vi "Proceed.vi"(7 "component is ready (Y)":bool=TRUE, 8 "error in (no error)":errorcluster, 10 "ProceedMessage":refnum<class "ProceedMessage.lvclass">, 11 "Retiga in":refnum<class "Retiga.lvclass">) -> (0 "error out":errorcluster, 2 "all observers are ready?":bool, 3 "Retiga out":refnum<class "Retiga.lvclass">)   [LabVIEW 2012, in "Retiga.lvclass"]
doc: "The Proceed method is used to check if your component is ready. Also it checks if the observers are ready. When the observers and the component are ready, it sends the proceed to its observee. If it's the highest observee, it distributes a stop command."
uses:
  Retiga.lvclass
  <vilib>/Distrio/Murmex/ProceedMessage/ProceedMessage.lvclass
  Retiga.lvclass/Retiga.ctl
  <vilib>/Distrio/Murmex/GenericMessage/GenericMessage.lvclass
  <vilib>/Distrio/Murmex/Murmex/Murmex.lvclass
  <vilib>/Distrio/Murmex/Message/Add or replace parameter.vi
  <vilib>/Distrio/Murmex/Message/Message.lvclass
  <vilib>/vision/NI_Vision_Development_Module.lvlib
panel:
  out "loop time (ms)":u32
  # "This method is called when the PROCEED\ntrigger is sent. \n\nOverride this method when your component needs to\nrespond to this trigger. \n\nCall parent for proper implementation"
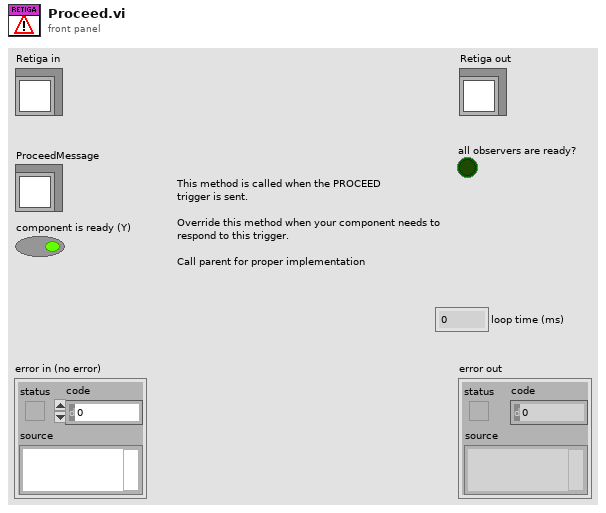
[diagram p1: front panel]
types:
  T1 = typedef "IMAQ Image.ctl" = refnum<image>
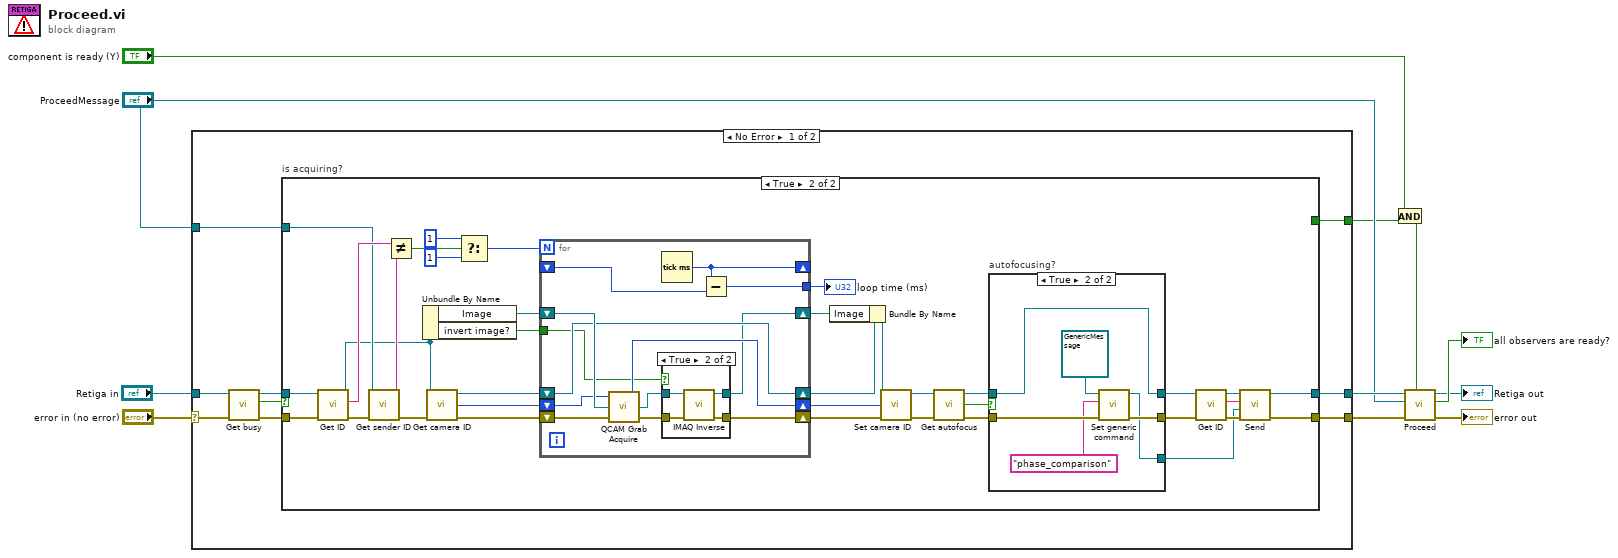
[diagram p0: block diagram]
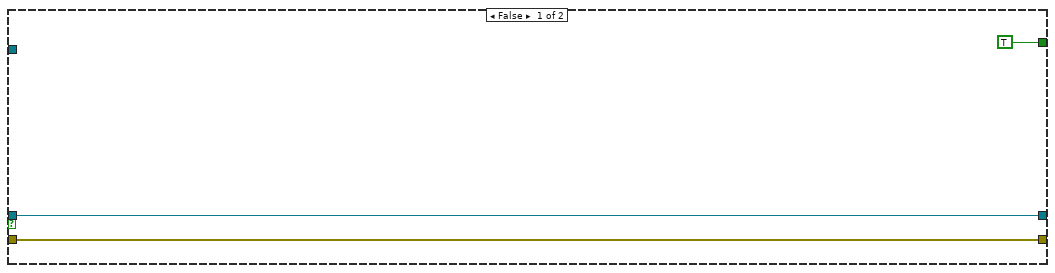
[diagram p2: hidden frame]
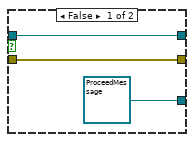
[diagram p3: hidden frame]
diagram:
  n1 = case shown="No Error" "error in (no error)" {
    selector: "error in (no error)" -> [w20 w89]
    tunnel: [w14 w89] -> w6
    tunnel: [w15 w88] -> w5
    tunnel: "Retiga in" -> [w19 w88]
    tunnel: "ProceedMessage" -> [w13 _]
    tunnel: [w12 _] -> w1
    frame No Error {
      n2 = call-dynamic "Get busy.vi"("error in (no error)"=w20, "Retiga in"=w19) -> ("error out"=w17:errorcluster, "busy?"=w18:bool, "Retiga out"=w16:refnum<class "Retiga.lvclass">)  [unwired: 7 in]
      n3 = case "is acquiring?" shown="True" w18 {
        tunnel: w17 -> [w22 w56]
        tunnel: w16 -> [w23 w55]
        tunnel: [w23 w27] -> w15
        tunnel: [w22 w26] -> w14
        tunnel: w13 -> [_ w54]
        tunnel: [TRUE _] -> w12
        frame False {
        }
        frame True {
          n4 = call <vilib>:"Get ID.vi"("error in (no error)"=w56, "Murmex in"=w55) -> ("error out"=w59:errorcluster, "component id"=w58:string, "Murmex out"=w48:refnum<class "Retiga.lvclass">)  [unwired: 7 in]
          n5 = call <vilib>:"Get sender ID.vi"("error in (no error)"=w59, "Message in"=w54) -> ("error out"=w49:errorcluster, "sender"=w57:string)  [unwired: 7 in, 1 out]
          n6 = Not Equal?(x=w58, y=w57) -> (x != y?=w51:bool)
          n7 = Unbundle By Name(w48) -> ("Image"=w44:T1, "invert image?"=w24:bool)
          n8 = call-dynamic "Get camera ID.vi"("error in (no error)"=w49, "Retiga in"=w48) -> ("error out"=w46:errorcluster, "camera ID"=w45:u32, "Retiga out"=w47:refnum<class "Retiga.lvclass">)  [unwired: 7 in]
          n9 = Select(t=1, s=w51, f=1) -> (s? t:f=w50:i32)
          n10 = for {
            N: w50 -> [_]
            shift-right: [w77] -> w43
            shift-left: w47 -> [w77]
            shift-right: [w75] -> w40
            shift-left: w46 -> [w81]
            shift-right: [w78] -> w39
            shift-left: w45 -> [w79]
            shift-right: [w73] -> w42
            shift-left: w44 -> [w80]
            shift-right: [w71] -> _
            shift-left: _ -> [w72]
            tunnel: [w70] -> w25
            tunnel: w24 -> [w69]
            n11 = call <userlib>:"QCAM Grab Acquire.vi"("error in (no error)"=w81, "Image"=w80, "cameraId"=w79) -> ("error out"=w76:errorcluster, "Image Out"=w74:T1, "cameraId out"=w78:u32)
            n12 = Tick Count (ms)() -> (millisecond timer value=w71:u32)
            n13 = case shown="True" w69 {
              tunnel: w76 -> [w82 w87]
              tunnel: [w82 w86] -> w75
              tunnel: w74 -> [w83 w85]
              tunnel: [w83 w84] -> w73
              frame False {
              }
              frame True {
                n14 = call "IMAQ Inverse"("error in (no error)"=w87, "Image Src"=w85) -> ("error out"=w86:errorcluster, "Image Dst Out"=w84:T1)  [unwired: 8 in]
              }
            }
            n15 = Subtract(x=w71, y=w72) -> (x-y=w70:u32)
          }
          "loop time (ms)" <- w25
          n16 = Bundle By Name(cluster=w43, "Image"=w42) -> (w41:refnum<class "Retiga.lvclass">)
          n17 = call-dynamic "Set camera ID.vi"("error in (no error)"=w40, "camera ID"=w39, "Retiga in"=w41) -> ("error out"=w37:errorcluster, "Retiga out"=w38:refnum<class "Retiga.lvclass">)  [unwired: 7 in]
          n18 = call-dynamic "Get autofocus.vi"("error in (no error)"=w37, "Retiga in"=w38) -> ("error out"=w36:errorcluster, "autofocusing?"=w35:bool, "Retiga out"=w34:refnum<class "Retiga.lvclass">)  [unwired: 7 in]
          n19 = case "autofocusing?" shown="True" w35 {
            tunnel: [refnum<class "ProceedMessage.lvclass"> refnum ("Distrio Murmex 1.5:ProceedMessage") w66] -> w28
            tunnel: [w61 w67] -> w31
            tunnel: w36 -> [w61 w68]
            tunnel: w34 -> [w60 w65]
            tunnel: [w60 w65] -> w30
            frame False {
            }
            frame True {
              n20 = call <vilib>:"Set generic command.vi"("error in (no error)"=w68, "generic command"="phase_comparison", "GenericMessage in"=refnum<class "GenericMessage.lvclass"> refnum ("Message in")) -> ("error out"=w67:errorcluster, "GenericMessage out"=w66:refnum<class "GenericMessage.lvclass">)  [unwired: 7 in]
            }
          }
          n21 = call <vilib>:"Get ID.vi"("error in (no error)"=w31, "Murmex in"=w30) -> ("error out"=w29:errorcluster, "component id"=w32:string, "Murmex out"=w33:refnum<class "Retiga.lvclass">)  [unwired: 7 in]
          n22 = call <vilib>:"Send.vi"("error in (no error)"=w29, "Message"=w28, "recipient"=w32, "Murmex in"=w33) -> ("error out"=w26:errorcluster, "Murmex out"=w27:refnum<class "Retiga.lvclass">)  [unwired: 6 in]
        }
      }
    }
    frame Error {
    }
  }
  n23 = And(x="component is ready (Y)", y=w1) -> (x .and. y?=w2:bool)
  n24 = call-parent "Proceed.vi"("component is ready (Y)"=w2, "error in (no error)"=w6, "ProceedMessage"="ProceedMessage", "Murmex in"=w5) -> ("error out"=→"error out":errorcluster, "all observers are ready?"=→"all observers are ready?":bool, "Murmex out"=→"Retiga out":refnum<class "Retiga.lvclass">)  [unwired: 5 in]
